vi "String Match Between.vi"(8 "End String":string, 9 "Start String":string, 10 "Input String":string) -> (1 "Resultant String":string)   [LabVIEW 2011]
doc: "Returns the substring between two strings.\n\n<b>Input String</b> - String to search.\n\n<b>Start String</b> - String to find that designates the start of the string to find.\n\n<b>End String</b> - String to find that designates the end of the string to find.\n\nExample:\n<b>Input String:</b> This String has a comment /test/in it.\n<b>Start String:</b> /\n<b>End String:</b> /\n<b>Resultant String</b> test\n\n\nVersion 1.0 - 10/20/2009\n\nPhaeron, Inc.\nwww.phaeron.com\ninfo@phaeron.com"
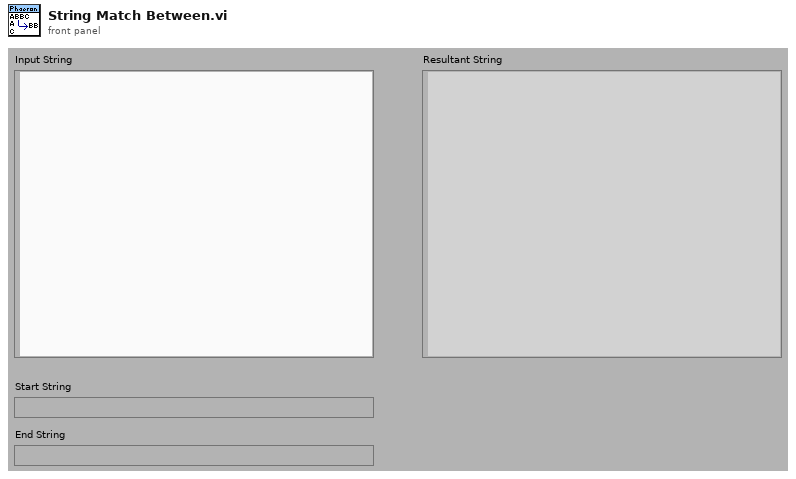
[diagram p1: front panel]
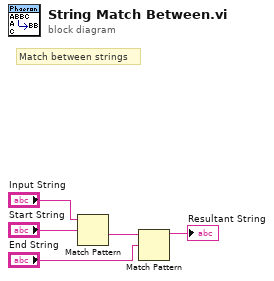
[diagram p0: block diagram]
diagram:
  # "Match between strings"
  n1 = Match Pattern(string="Input String", regular expression="Start String") -> (after substring=w5:string)  [unwired: 1 in, 3 out]
  n2 = Match Pattern(string=w5, regular expression="End String") -> (before substring=→"Resultant String":string)  [unwired: 1 in, 3 out]
